vi "NotifyWithoutDataOverride.vi"(8 "error in (no error)":errorcluster, 11 "TCP Com in":refnum<class "TCP Com.lvclass">) -> (0 "error out":errorcluster, 2 "Data out":refnum<class "Data.lvclass">, 3 "TCP Com out":refnum<class "TCP Com.lvclass">)   [LabVIEW 2023, in "TCP Com.lvclass"]
uses:
  TCP Com.lvclass
  Data/Data.lvclass
  TCP Com.lvclass/TCP Com.ctl
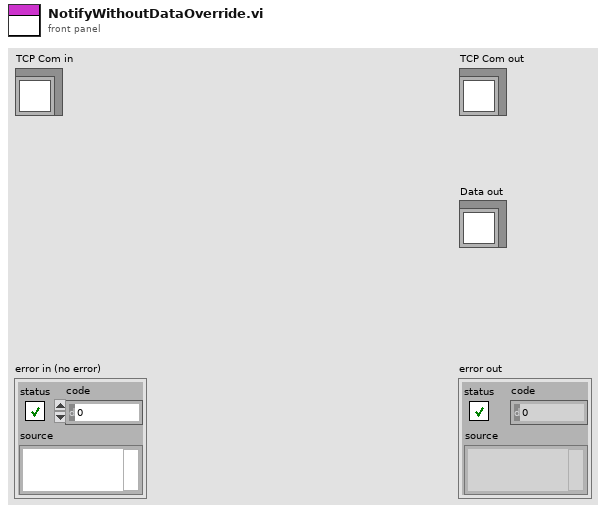
[diagram p1: front panel]
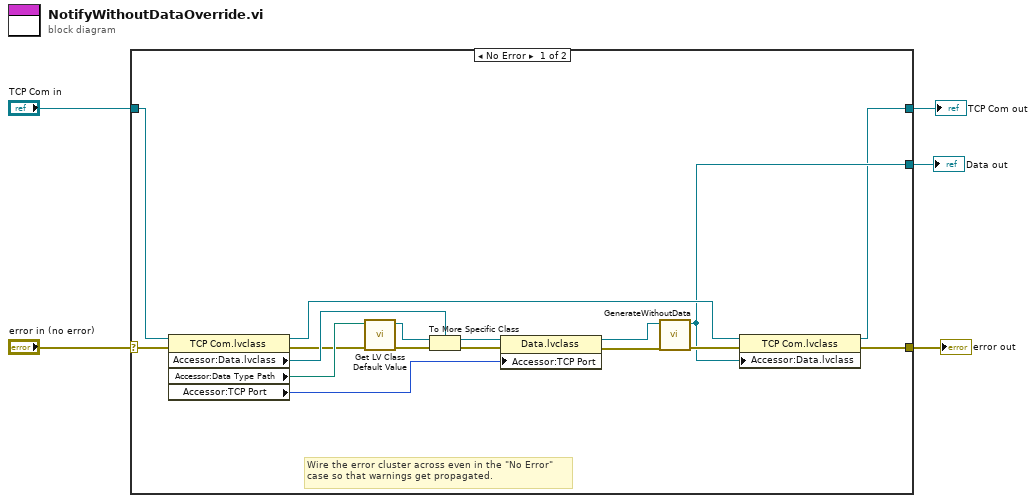
[diagram p0: block diagram]
diagram:
  n1 = case shown="No Error" "error in (no error)" {
    selector: "error in (no error)" -> [w9 w24]
    tunnel: [w8 w24] -> w4
    tunnel: [w6 w23] -> w2
    tunnel: "TCP Com in" -> [w10 w23]
    tunnel: [w7 _] -> w1
    frame No Error {
      # "Wire the error cluster across even in the \"No Error\"\ncase so that warnings get propagated."
      n2 = property class="TCP Com.lvclass"(reference=w10, error in=w9) -> (reference out=w15:refnum<class "TCP Com.lvclass">, error out=w17:errorcluster, "Accessor:Data.lvclass"=w19:refnum<class "Data.lvclass">, "Accessor:Data Type Path"=w18:path, "Accessor:TCP Port"=w11:u16)
      n3 = call <vilib>:"Get LV Class Default Value.vi"("error in (no error)"=w17, "class path"=w18) -> ("error out"=w22:errorcluster, "object"=w21:refnum<class>)  [unwired: 8 in]
      n4 = To More Specific Class(target class=w19, reference=w21, error in=w22) -> (specific class reference=w20:refnum<class "Data.lvclass">, error out=w13:errorcluster)
      n5 = property class="Data.lvclass"(reference=w20, error in=w13, "Accessor:TCP Port"=w11) -> (reference out=w14:refnum<class "Data.lvclass">, error out=w12:errorcluster)
      n6 = call-dynamic "GenerateWithoutData.vi"("error in (no error)"=w12, "Data in"=w14) -> ("error out"=w16:errorcluster, "Data out"=w7:refnum<class "Data.lvclass">)  [unwired: 8 in]
      n7 = property class="TCP Com.lvclass"(reference=w15, error in=w16, "Accessor:Data.lvclass"=w7) -> (reference out=w6:refnum<class "TCP Com.lvclass">, error out=w8:errorcluster)
    }
    frame Error {
    }
  }
  "error out" <- w4
  "TCP Com out" <- w2
  "Data out" <- w1
